vi "Quat_to_PRY.vi"(1 "toDegrees? (T)":bool=TRUE, 2 "Quaternion":cluster{"x":dbl, "y":dbl, "z":dbl, "w":dbl}) -> (0 "Orientation":T1)   [LabVIEW 2014]
doc: "Converts a Quaternion to Pitch, Roll, Yaw orientation."
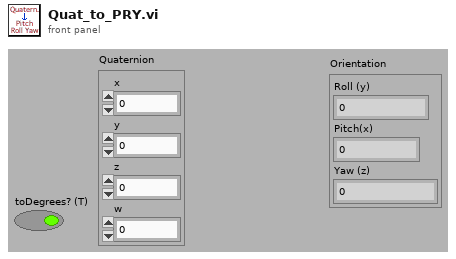
[diagram p1: front panel]
types:
  T1 = cluster{"Roll (y)":dbl, "Pitch(x)":dbl, "Yaw (z)":dbl}
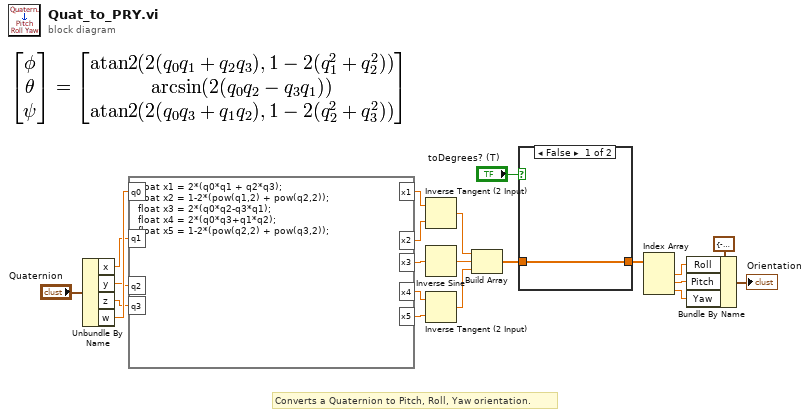
[diagram p0: block diagram]
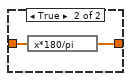
[diagram p2: hidden frame]
diagram:
  # "Converts a Quaternion to Pitch, Roll, Yaw orientation."
  n1 = Unbundle By Name("Quaternion") -> ("x"=w20:dbl, "y"=w19:dbl, "z"=w18:dbl, "w"=w21:dbl)
  n2 = formula code="float x1 = 2*(q0*q1 + q2*q3);\nfloat x2 = 1-2*(pow(q1,2) + pow(q2,2));\nfloat x3 = 2*(q0*q2-q3*q1);\nfloat x4 = 2*(q0*q3+q1*q2);\nfloat x5 = 1-2*(pow(q2,2) + pow(q3,2));"("q0"=w21, "q1"=w20, "q2"=w19, "q3"=w18) -> ("x1"=w17:dbl, "x2"=w16:dbl, "x3"=w13:dbl, "x4"=w15:dbl, "x5"=w14:dbl)
  n3 = Inverse Tangent (2 Input)(1:w16, 2:w17) -> (0:w12:dbl)
  n4 = Inverse Sine(1:w13) -> (0:w11:dbl)
  n5 = Inverse Tangent (2 Input)(1:w14, 2:w15) -> (0:w10:dbl)
  n6 = Build Array(w12, w11, w10) -> (w9:dbl[])
  n7 = case shown="False" "toDegrees? (T)" {
    tunnel: w9 -> [w22 w24]
    tunnel: [w22 w23] -> w8
    frame False {
    }
    frame True {
      n8 = expression code="x*180/pi"(w24) -> (w23:dbl[])
    }
  }
  n9 = Index Array(array=w8) -> (element #1=w5:dbl, element #2=w4:dbl, element #3=w3:dbl)  [unwired: 3 in]
  n10 = Bundle By Name(cluster=cluster{"Roll":dbl, "Pitch":dbl, "Yaw":dbl} {"Roll"=-22.96953055973984, "Pitch"=0.09723239880810781, "Yaw"=-0.35868840863814605} ("Orientation"), "Roll"=w5, "Pitch"=w4, "Yaw"=w3) -> (→"Orientation":cluster{"Roll":dbl, "Pitch":dbl, "Yaw":dbl})
